vi "Main.vi"(0 "Proto File Path":path[](array[path]), 1 "Generated Library Name":string, 2 "Generate":enum16{"gRPC Server", "gRPC Client", "Both"}(ring), 5 "Import Paths":path[](array[path]), 7 "Prototype Library":path, 9 "Target Project":path, 11 "Target Name":string, 12 "Library Suffix":string caption="Generated Library Suffix (\"_server\" / \"_client\" will be added by default)") -> ()   [LabVIEW 2019, in "gRPC Template Creation Utility.lvlib"]
uses:
  gRPC Template Creation Utility.lvlib
  TypeDefs/Project Settings.ctl
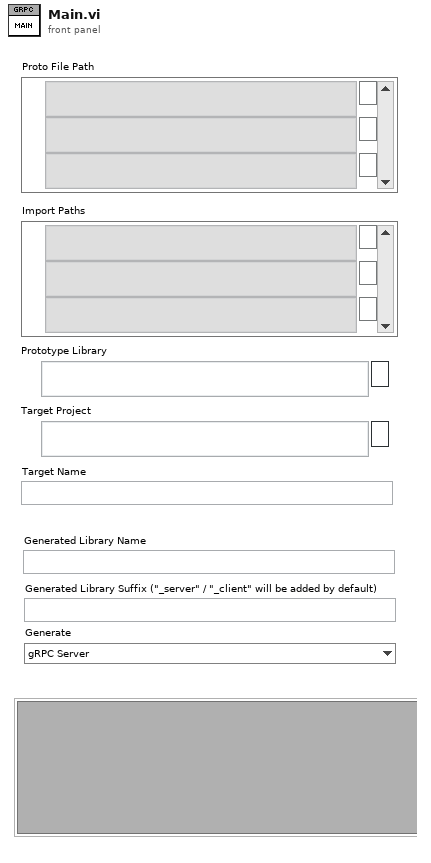
[diagram p1: front panel]
types:
  T1 = typedef "gRPC Template Creation Utility.lvlib/RPC Method Parameters.ctl" = cluster{"RPC Method Name":string, "Request Metadata Name":string, "Response Metadata Name":string, "Client Streaming":bool, "Server Streaming":bool}
  T2 = typedef "gRPC Template Creation Utility.lvlib/Enum Metadata (Scripting).ctl" = cluster{"Version":i32, "Name":string, "Type Url":string, "Enum Values":string, "Allow Alias":bool}
  T3 = typedef "gRPC Template Creation Utility.lvlib/Message Metadata (Scripting).ctl" = cluster{"Version":i32, "Name":string, "Type Url":string, "Elements":T4[]}
  T4 = typedef "gRPC Template Creation Utility.lvlib/Message Element Metadata (Scripting).ctl" = cluster{"Field Name":string, "Embedded Message Name":string, "Protobuf Index":i32, "MessageElementType":T5, "Repeated":bool}
  T5 = typedef "gRPC Template Creation Utility.lvlib/Message Element Type.ctl" = enum32{"Int32Value", "FloatValue", "DoubleValue", "BoolValue", "StringValue", "MessageValue", "Int64Value", "UInt32Value", "UInt64Value", "EnumValue", "Bytes", "Fixed64", "Fixed32", "SFixed64", "SFixed32", "SInt64", "SInt32", "Oneof"}
  T6 = typedef "gRPC Template Creation Utility.lvlib/Oneof Metadata.ctl" = cluster{"Version":i32, "Name":string, "Elements":T4[], "Selected Field":string}
  T7 = typedef "gRPC Template Creation Utility.lvlib/Project Settings.ctl" = cluster{"Target Project Path":path, "Target Name":string, "Server Name":string, "Library Path":path}
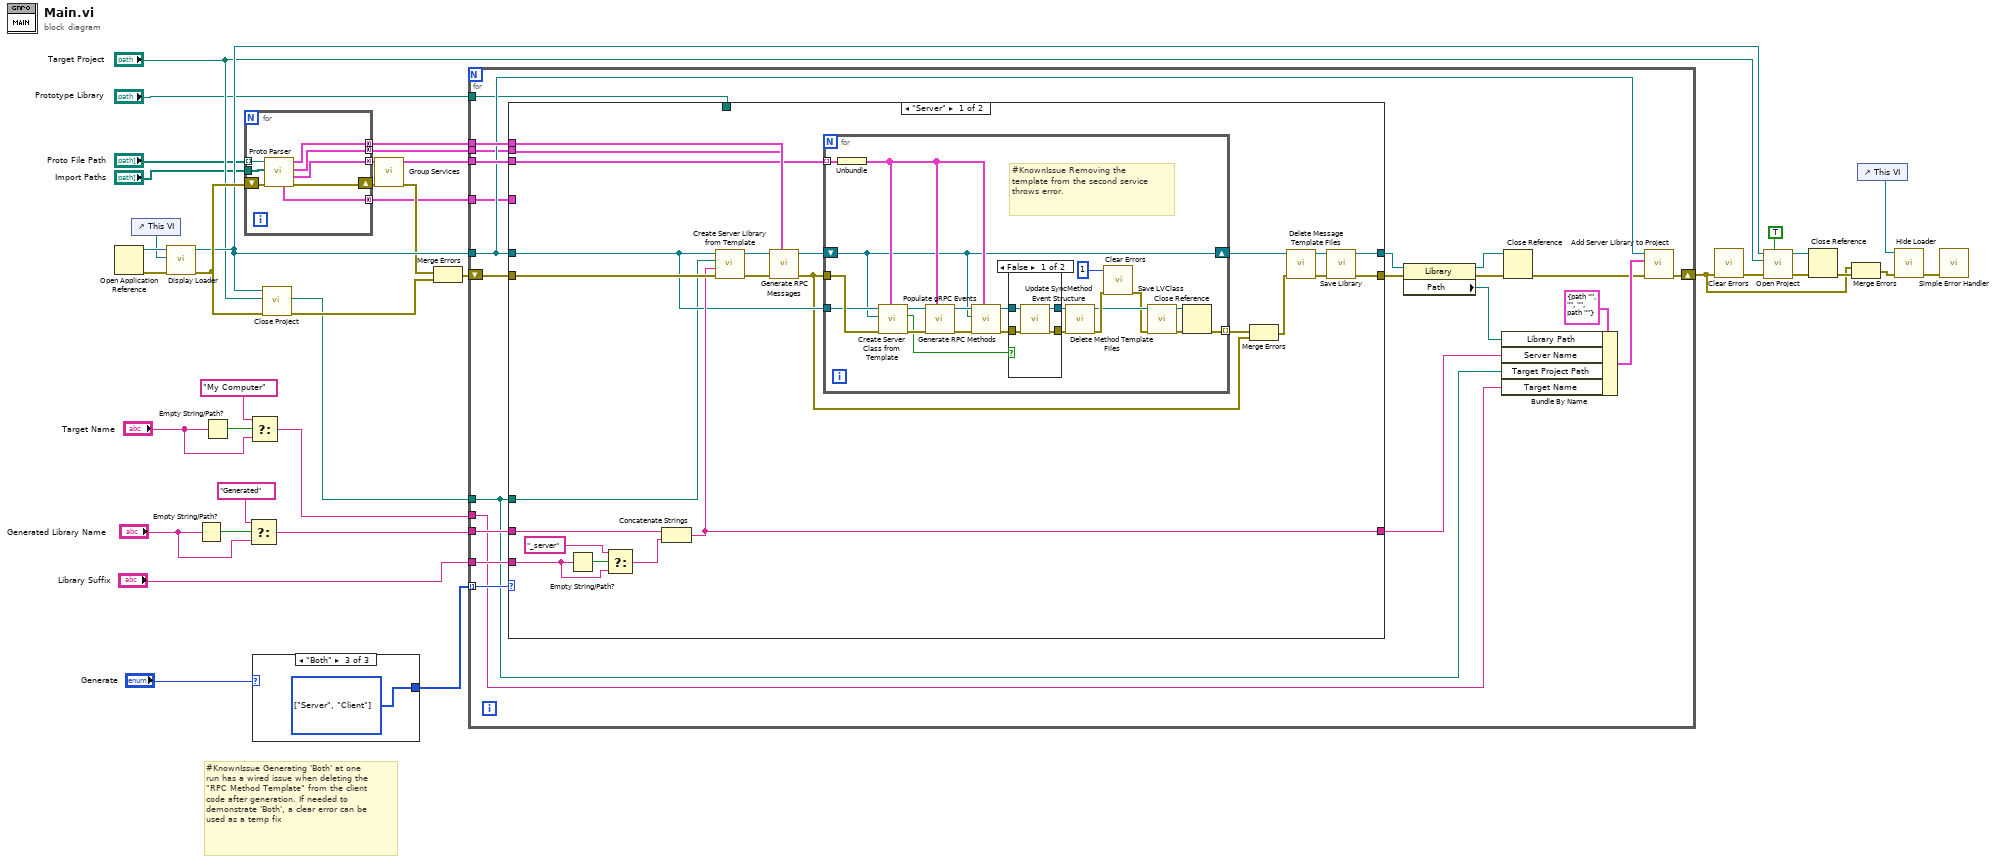
[diagram p0: block diagram]
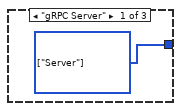
[diagram p2: hidden frame]
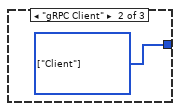
[diagram p3: hidden frame]
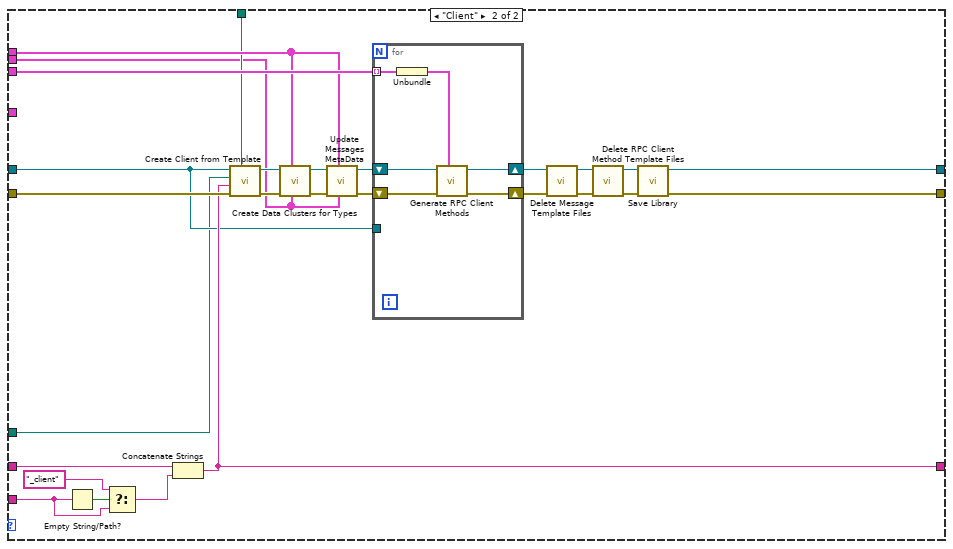
[diagram p5: hidden frame]
diagram:
  # "#KnownIssue Generating 'Both' at one run has a wired issue when deleting the \"RPC Method Template\" from the client code after generation. If needed to demonstrate 'Both', a clear error can be used as a temp fix"
  n1 = Open Application Reference() -> (0:w32:errorcluster, 3:w31:refnum<vi>)  [unwired: 4 in]
  n2 = control-ref of="This VI"() -> (w29:refnum<vi>)
  n3 = call "Display Loader.vi"("error in (no error)"=w32, "VI in"=w29, "application ref in"=w31) -> ("error out"=w30:errorcluster, "application ref out"=w17:refnum<vi>)  [unwired: 7 in]
  n4 = Empty String/Path?(string/path="Generated Library Name") -> (empty?=w39:bool)
  n5 = Empty String/Path?(string/path="Target Name") -> (empty?=w24:bool)
  n6 = for {
    tunnel: [w42] -> w34 mode=concatenating
    tunnel: [w46] -> w7 mode=concatenating
    shift-right: [w47] -> w9
    shift-left: w30 -> [w45]
    tunnel: "Proto File Path" -> [w44] mode=indexing
    tunnel: "Import Paths" -> [w43]
    tunnel: [w41] -> w2 mode=concatenating
    tunnel: [w40] -> w1 mode=concatenating
    n7 = call "Proto Parser.vi"("error in (no error)"=w45, "Import Paths"=w43, ".proto file path"=w44) -> ("error out"=w47:errorcluster, "gRPC Method Parameters"=w46:T1[], "gRPC Enum Parameters"=w41:T2[], "gRPC Message Parameters"=w42:T3[], "gRPC Oneof Parameters"=w40:T6[])  [unwired: 4 in]
  }
  n8 = Select(t="Generated" ("Path"), s=w39, f="Generated Library Name") -> (s? t:f=w26:string)
  n9 = Select(t="My Computer" ("Path"), s=w24, f="Target Name") -> (s? t:f=w22:string)
  n10 = case shown="\"Both\"" "Generate" {
    tunnel: [w48 w49 w50] -> w21
    frame "gRPC Server" {
      w48 = enum16{"Server", "Client"}[] [enum."Server"] items=["Server", "Client"]
    }
    frame "gRPC Client" {
      w49 = enum16{"Server", "Client"}[] [enum."Client"] items=["Server", "Client"]
    }
    frame "Both" {
      w50 = enum16{"Server", "Client"}[] [enum."Server", enum."Client"] items=["Server", "Client"]
    }
  }
  n11 = call "Close Project.vi"("error in (no error)"=w30, "Project Path in"="Target Project", "Application reference"=w17) -> ("error out"=w36:errorcluster, "Project Path out"=w27:path)  [unwired: 6 in, 1 out]
  n12 = call "Group Services.vi"("error in"=w9, "gRPC Method Parameters"=w7) -> ("error out"=w8:errorcluster, "Service Methods"=w6:cluster{"gRPC Method Parameters":T1[]}[])  [unwired: 8 in]
  n13 = Merge Errors(w8, w36) -> (w35:errorcluster)
  n14 = for {
    tunnel: w34 -> [w71]
    tunnel: w6 -> [w70]
    tunnel: w27 -> [w55]
    tunnel: w26 -> [w63]
    tunnel: w22 -> [w54]
    tunnel: w17 -> [w61]
    shift-right: [w58] -> w11
    shift-left: w35 -> [w72]
    tunnel: w21 -> [w57] mode=indexing
    tunnel: "Library Suffix" -> [w56]
    tunnel: "Prototype Library" -> [w53]
    tunnel: w2 -> [w52]
    tunnel: w1 -> [w51]
    n15 = case shown="\"Server\"" w57 {
      tunnel: w72 -> [w95 w149]
      tunnel: w71 -> [w94 w138]
      tunnel: w70 -> [w93 w148]
      tunnel: [w92 w147] -> w69
      tunnel: [w74 w135] -> w67
      tunnel: w63 -> [w91 w146]
      tunnel: [w90 w145] -> w62
      tunnel: w61 -> [w89 w144]
      tunnel: w55 -> [w88 w143]
      tunnel: w56 -> [w77 w130]
      tunnel: w53 -> [_ w128]
      tunnel: w52 -> [w76 w127]
      tunnel: w51 -> [_ _]
      frame "Server" {
        n16 = Empty String/Path?(string/path=w77) -> (empty?=w80:bool)
        n17 = Select(t="_server" ("string"), s=w80, f=w77) -> (s? t:f=w78:string)
        n18 = Concatenate Strings(w91, w78) -> (w90:string)
        n19 = call "Create Server Library from Template.vi"("error in (no error)"=w95, "Generated Server Name"=w90, "Target Project Path"=w88, "Application ref in"=w89) -> ("error out"=w86:errorcluster, "Server library out"=w87:refnum<vi>)  [unwired: 6 in]
        n20 = call "Generate RPC Messages.vi"("Enum Metadata"=w76, "Messages Metadata"=w94, "error in (no error)"=w86, "Library"=w87) -> ("error out"=w73:errorcluster, "Library"=w85:refnum<vi>)  [unwired: 6 in]
        n21 = for {
          tunnel: w93 -> [w114] mode=indexing
          shift-right: [w105] -> w84
          shift-left: w85 -> [w105]
          tunnel: w89 -> [w115]
          tunnel: w73 -> [w116]
          tunnel: [w111] -> w83 mode=indexing
          # "#KnownIssue Removing the template from the second service throws error."
          n22 = Unbundle(w114) -> ("gRPC Method Parameters"=w106:T1[])
          n23 = call "Create Server Class from Template.vi"("gRPC Method Parameters"=w106, "error in (no error)"=w116, "Library"=w105, "Application ref in"=w115) -> ("error out"=w109:errorcluster, "Already Exists ?"=w100:bool, "LVClassLibrary in"=w110:refnum<vi>)  [unwired: 5 in]
          n24 = call "Populate gRPC Events.vi"("RPC Method Parameters"=w106, "error in (no error)"=w109, "Server class in"=w110) -> ("error out"=w107:errorcluster, "Server class out"=w108:refnum<vi>)  [unwired: 7 in]
          n25 = call "Generate RPC Methods.vi"("RPC Method Parameters"=w106, "error in (no error)"=w107, "Library"=w105, "Server class in"=w108) -> ("error out"=w102:errorcluster, "Server class out"=w104:refnum<vi>)  [unwired: 6 in]
          n26 = case shown="False" w100 {
            tunnel: w104 -> [w120 w122]
            tunnel: [w119 w122] -> w103
            tunnel: w102 -> [w118 w121]
            tunnel: [w117 w121] -> w101
            frame False {
              n27 = call "Update SyncMethod Event Structure.vi"("error in (no error)"=w118, "Server class in"=w120) -> ("error out"=w117:errorcluster, "Server class out"=w119:refnum<vi>)  [unwired: 8 in]
            }
            frame True {
            }
          }
          n28 = call "Delete Method Template Files.vi"("error in (no error)"=w101, "LVClassLibrary in"=w103) -> ("error out"=w98:errorcluster, "LVClassLibrary out"=w97:refnum<vi>)  [unwired: 8 in]
          n29 = call <vilib>:"Clear Errors.vi"("error in (no error)"=w98, "specific error code to clear (0: all)"=1) -> ("error out"=w96:errorcluster)  [unwired: 4 in, 1 out]
          n30 = call "Save LVClass.vi"("error in (no error)"=w96, "LVClassLibrary in"=w97) -> ("error out"=w113:errorcluster, "LVClassLibrary out"=w112:refnum<vi>)  [unwired: 8 in]
          n31 = Close Reference(reference=w112, error in (no error)=w113) -> (error out=w111:errorcluster)
        }
        n32 = Merge Errors(w83, w73) -> (w75:errorcluster)
        n33 = call "Delete Message Template Files.vi"("error in (no error)"=w75, "Library"=w84) -> ("error out"=w82:errorcluster, "Library"=w81:refnum<vi>)  [unwired: 8 in]
        n34 = call "Save Library.vi"("error in (no error)"=w82, "Library in"=w81) -> ("error out"=w74:errorcluster, "Library out"=w92:refnum<vi>)  [unwired: 8 in]
      }
      frame "Client" {
        n35 = Empty String/Path?(string/path=w130) -> (empty?=w132:bool)
        n36 = Select(t="_client" ("string"), s=w132, f=w130) -> (s? t:f=w129:string)
        n37 = Concatenate Strings(w146, w129) -> (w145:string)
        n38 = call "Create Client from Template.vi"("Template Library"=w128, "error in (no error)"=w149, "Generated Server Name"=w145, "Target Project Path"=w143, "Application ref in"=w144) -> ("error out"=w142:errorcluster, "Server library out"=w141:refnum<vi>)  [unwired: 5 in]
        n39 = call "Create Data Clusters for Types.vi"("Enum parameters"=w127, "Message parameters"=w138, "error in (no error)"=w142, "Library in"=w141) -> ("error out"=w140:errorcluster, "Library out"=w139:refnum<vi>)  [unwired: 6 in]
        n40 = call "Update Messages MetaData.vi"("Enum MetaData"=w127, "Messages MetaData"=w138, "error in (no error)"=w140, "Library"=w139) -> ("error out"=w137:errorcluster, "Library"=w136:refnum<vi>)  [unwired: 6 in]
        n41 = for {
          tunnel: w148 -> [w155] mode=indexing
          shift-right: [w150] -> w125
          shift-left: w136 -> [w152]
          tunnel: w144 -> [_]
          shift-right: [w151] -> w126
          shift-left: w137 -> [w153]
          n42 = Unbundle(w155) -> ("gRPC Method Parameters"=w154:T1[])
          n43 = call "Generate RPC Client Methods.vi"("RPC Method Parameters"=w154, "error in (no error)"=w153, "Library"=w152) -> ("error out"=w151:errorcluster, "Library"=w150:refnum<vi>)  [unwired: 7 in]
        }
        n44 = call "Delete Message Template Files.vi"("error in (no error)"=w126, "Library"=w125) -> ("error out"=w123:errorcluster, "Library"=w124:refnum<vi>)  [unwired: 8 in]
        n45 = call "Delete RPC Client Method Template Files.vi"("error in (no error)"=w123, "Library"=w124) -> ("error out"=w133:errorcluster, "Library"=w134:refnum<vi>)  [unwired: 8 in]
        n46 = call "Save Library.vi"("error in (no error)"=w133, "Library in"=w134) -> ("error out"=w135:errorcluster, "Library out"=w147:refnum<vi>)  [unwired: 8 in]
      }
    }
    n47 = property class="Library"(reference=w69, error in=w67) -> (reference out=w68:refnum<vi>, error out=w60:errorcluster, "Path"=w65:path)
    n48 = Bundle By Name(cluster=T7 {"Target Project Path"=path "", "Target Name"="", "Server Name"="", "Library Path"=path ""} ("Project Settings"), "Library Path"=w65, "Server Name"=w62, "Target Project Path"=w55, "Target Name"=w54) -> (w64:T7)
    n49 = Close Reference(reference=w68, error in (no error)=w60) -> (error out=w59:errorcluster)
    n50 = call "Add Server Library to Project.vi"("error in (no error)"=w59, "Project Settings"=w64, "Application in"=w61) -> ("error out"=w58:errorcluster)  [unwired: 8 in]
  }
  n51 = call <vilib>:"Clear Errors.vi"("error in (no error)"=w11) -> ("error out"=w13:errorcluster)  [unwired: 5 in, 1 out]
  n52 = call "Open Project.vi"("Open Project Window ?"=TRUE, "error in (no error)"=w13, "Project Path in"="Target Project", "Application reference"=w17) -> ("error out"=w15:errorcluster, "Application out"=w16:refnum<vi>)  [unwired: 5 in, 1 out]
  n53 = Close Reference(reference=w16, error in (no error)=w15) -> (error out=w19:errorcluster)
  n54 = Merge Errors(w11, w19) -> (w12:errorcluster)
  n55 = control-ref of="This VI"() -> (w33:refnum<vi>)
  n56 = call "Hide Loader.vi"("error in (no error)"=w12, "VI in"=w33) -> ("error out"=w28:errorcluster)  [unwired: 9 in]
  n57 = call <vilib>:"Simple Error Handler.vi"("error in (no error)"=w28) -> ()  [unwired: 4 in, 5 out]
